vi "Initialize Instrument.vi"(8 "error in (no error)":errorcluster, 10 "Reset":bool, 11 "HP 3457A in":refnum<class "HP 3457A.lvclass">) -> (0 "error out":errorcluster, 3 "HP 3457A out":refnum<class "HP 3457A.lvclass">)   [LabVIEW 2020, in "HP 3457A.lvclass"]
uses:
  HP 3457A.lvclass
  C:/Sandbox/Git_Sandbox/WiSpry Test Framework source code (LV20)/WiSpry Test Framework/Instruments/Instrument.lvclass
  Instrument.lvclass/Instrument.ctl
  Digital Multimeter.lvclass
  Instrument.lvclass
panel:
  out "return count":u32
  out "read buffer":string
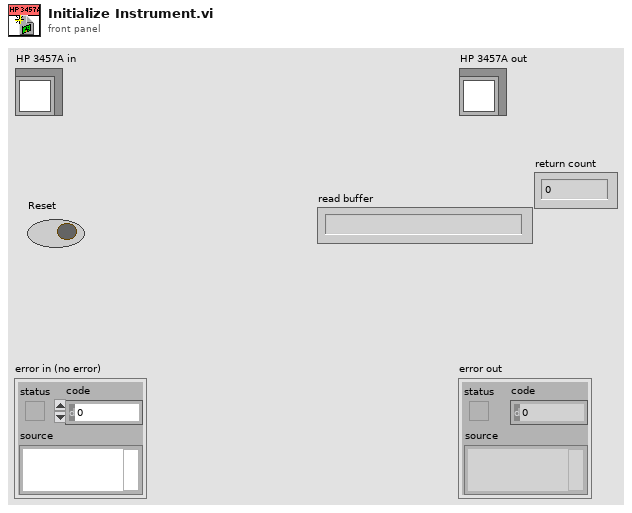
[diagram p1: front panel]
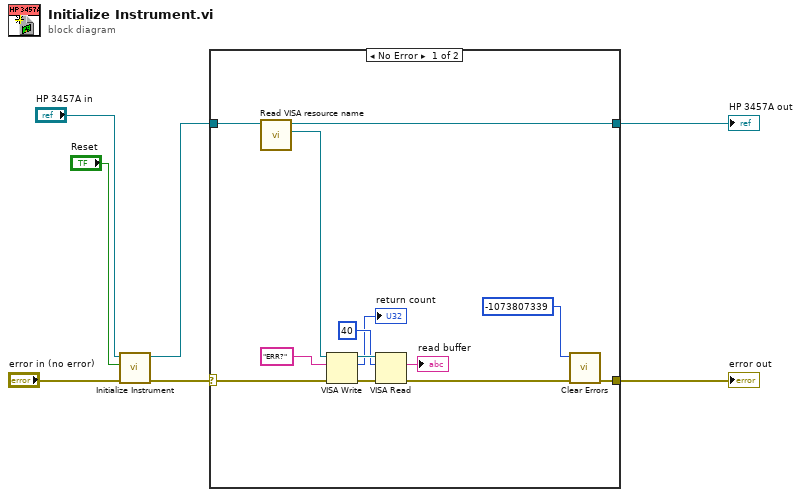
[diagram p0: block diagram]
diagram:
  n1 = call-parent "Initialize Instrument.vi"("error in (no error)"="error in (no error)", "Reset"="Reset", "Instrument in"="HP 3457A in") -> ("error out"=w4:errorcluster, "Instrument out"=w3:refnum<class "HP 3457A.lvclass">)  [unwired: 7 in]
  n2 = case shown="No Error" w4 {
    selector: w4 -> [w13 w22]
    tunnel: w3 -> [w20 w21]
    tunnel: [w8 w22] -> w1
    tunnel: [w19 w21] -> w2
    frame No Error {
      n3 = call "Read VISA resource name.vi"("Instrument in"=w20) -> ("VISA resource name"=w12:refnum<visa-resource-name>, "Instrument out"=w19:refnum<class "HP 3457A.lvclass">)  [unwired: 9 in]
      n4 = VISA Write(VISA resource name=w12, write buffer="ERR?", error in (no error)=w13) -> (VISA resource name out=w18:refnum<visa-resource-name>, return count=→"return count":u32, error out=w17:errorcluster)
      n5 = VISA Read(VISA resource name=w18, byte count=u32 40, error in (no error)=w17) -> (read buffer=→"read buffer":string, error out=w9:errorcluster)  [unwired: 2 out]
      n6 = call <vilib>:"Clear Errors.vi"("error in (no error)"=w9, "specific error code to clear (0: all)"=-1073807339) -> ("error out"=w8:errorcluster)  [unwired: 4 in, 1 out]
    }
    frame Error {
    }
  }
  "error out" <- w1
  "HP 3457A out" <- w2
